vi "Node.Table.Get.vi"(8 "error in (no error)":errorcluster, 11 "Node":refnum<k24>) -> (0 "error out":errorcluster, 1 "Values":dbl[](array[numeric]), 2 "Names":string[](array[string]), 3 "Node out":refnum<k24>)   [LabVIEW 2015, in "Workspace.Obejct.Radio.lvlib"]
uses:
  NationalInstruments.VeriStand.SystemStorage
  Workspace.Obejct.Radio.lvlib
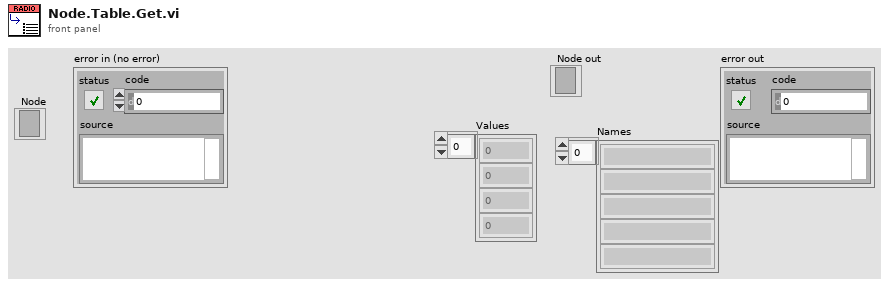
[diagram p1: front panel]
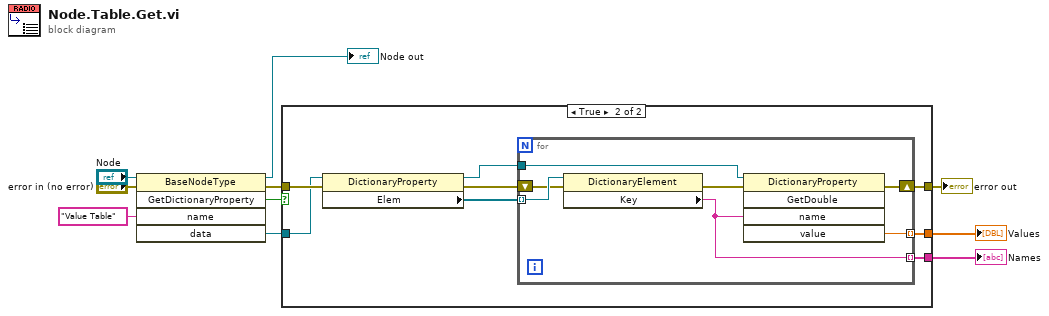
[diagram p0: block diagram]
diagram:
  n1 = invoke class="BaseNodeType" method="GetDictionaryProperty"(reference="Node", error in="error in (no error)", "name"="Value Table") -> (reference out=→"Node out":refnum<k24>, error out=w7:errorcluster, "GetDictionaryProperty"=w4:bool, "data"=w5:refnum<k24>)  [unwired: 2 in, 1 out]
  n2 = case shown="True" w4 {
    tunnel: [_ w18] -> w9
    tunnel: [_ w17] -> w8
    tunnel: w7 -> [w11 w16]
    tunnel: w5 -> [_ w14]
    tunnel: [w11 w12] -> w3
    frame False {
    }
    frame True {
      n3 = property class="DictionaryProperty"(reference=w14, error in=w16) -> (reference out=w13:refnum<k24>, error out=w15:errorcluster, "Elem"=w19:refnum<k24>[])
      n4 = for {
        tunnel: w19 -> [w26] mode=indexing
        tunnel: [w24] -> w18 mode=indexing
        tunnel: w13 -> [w25]
        tunnel: [w23] -> w17 mode=indexing
        shift-right: [w20] -> w12
        shift-left: w15 -> [w22]
        n5 = property class="DictionaryElement"(reference=w26, error in=w22) -> (error out=w21:errorcluster, "Key"=w24:string)  [unwired: 1 out]
        n6 = invoke class="DictionaryProperty" method="GetDouble"(reference=w25, error in=w21, "name"=w24) -> (error out=w20:errorcluster, "value"=w23:dbl)  [unwired: 2 in, 3 out]
      }
    }
  }
  "Names" <- w9
  "Values" <- w8
  "error out" <- w3
